vi "Enqueue Logs Element.vi"(8 "Error In":errorcluster, 9 "Timeout":i32, 10 "Event Occured":refnum<class "EventsAbstract.lvclass">, 11 "EventLog in":refnum<class "LogsAbstract.lvclass">) -> (0 "Error Out":errorcluster, 1 "Timed out?":bool, 3 "EventLog out":refnum<class "LogsAbstract.lvclass">)   [LabVIEW 2019, in "LogsAbstract.lvlib" / "LogsAbstract.lvclass"]
uses:
  LogsAbstract.lvclass
  Classes/EventsAbstract/EventsAbstract.lvclass
  Classes/Event/Event.lvclass
  C:/Projekty/_Wewnetrzne/PC_ActorFramework/07_Program/LABVIEW/02_Source/Classes/EventsAbstract/EventsAbstract.lvclass
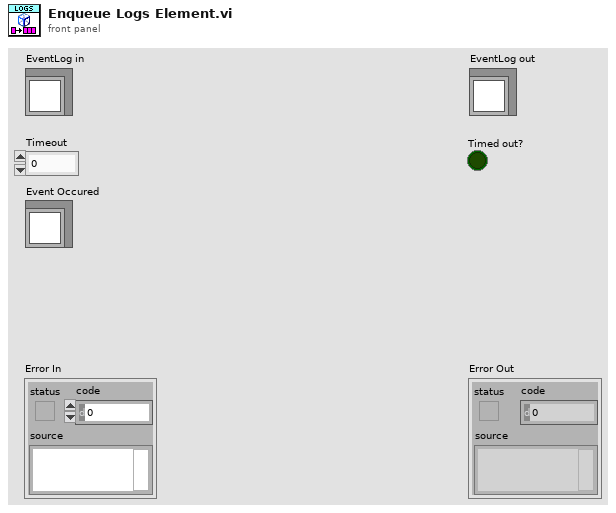
[diagram p1: front panel]
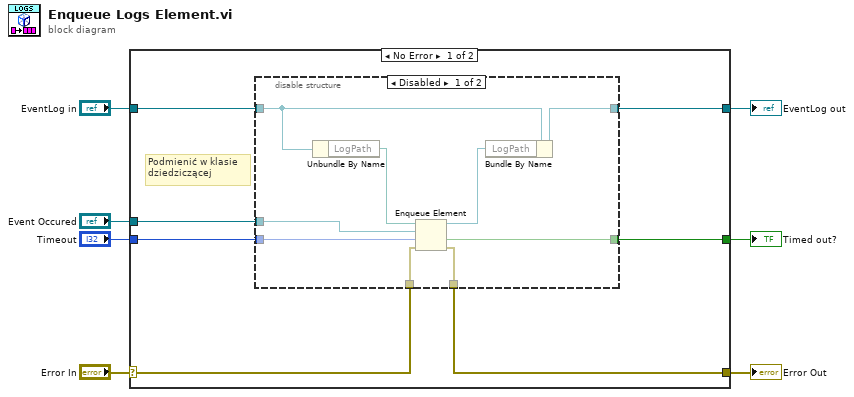
[diagram p0: block diagram]
diagram:
  n1 = case shown="No Error" "Error In" {
    selector: "Error In" -> [w13 w26]
    tunnel: [w9 w26] -> w6
    tunnel: [w12 w25] -> w4
    tunnel: "EventLog in" -> [w14 w25]
    tunnel: [w10 _] -> w3
    tunnel: "Timeout" -> [w11 _]
    tunnel: "Event Occured" -> [w8 _]
    frame No Error {
      # "Podmienić w klasie\ndziedziczącej"
      n2 = disable-structure shown="Disabled" {
        disable-tunnel: w14 -> [w23 w24]
        disable-tunnel: w13 -> [w21 _]
        disable-tunnel: [w20 w24] -> w12
        disable-tunnel: w11 -> [w18 _]
        disable-tunnel: [w17 _] -> w10
        disable-tunnel: [w16 _] -> w9
        disable-tunnel: w8 -> [w15 _]
        frame Disabled {
          n3 = Unbundle By Name(w23) -> ("LogPath"=w22:path)
          n4 = Enqueue Element(queue=w22, element=w15, timeout in ms (-1)=w18, error in (no error)=w21) -> (queue out=w19:refnum<queue>, timed out?=w17:bool, error out=w16:errorcluster)
          n5 = Bundle By Name(cluster=w23, "LogPath"=w19) -> (w20:refnum<class "LogsAbstract.lvclass">)
        }
        frame Enabled {
        }
      }
    }
    frame Error {
    }
  }
  "Error Out" <- w6
  "EventLog out" <- w4
  "Timed out?" <- w3
